vi "Test_StopWatch.vi"() -> ()   [LabVIEW 2018]
panel:
  in  "File":bool
  out "履歴":T1(array[cluster])
  out "FromLap":u32
  out "FromStart":u32
  in  "Lap":bool
  in  "Start":bool
  in  "停止":bool
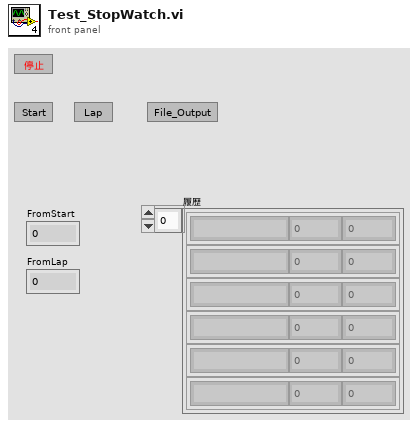
[diagram p1: front panel]
types:
  T1 = cluster{"Point":string, "FromLap":u32, "FromStart":u32}[]
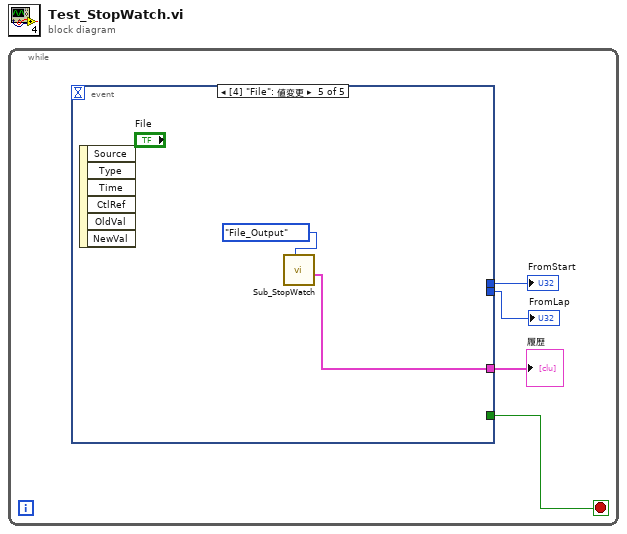
[diagram p0: block diagram]
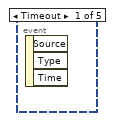
[diagram p2: hidden frame]
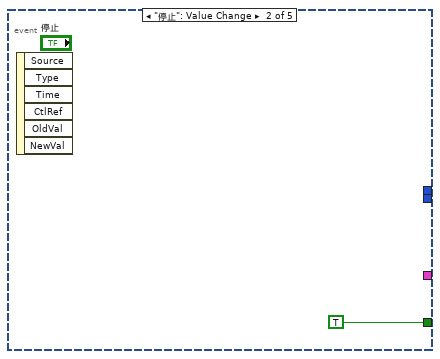
[diagram p3: hidden frame]
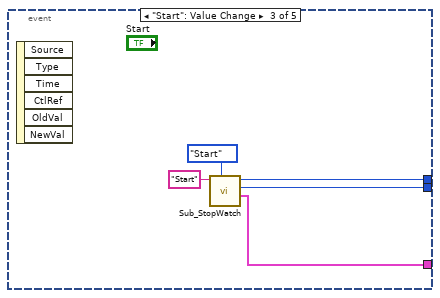
[diagram p4: hidden frame]
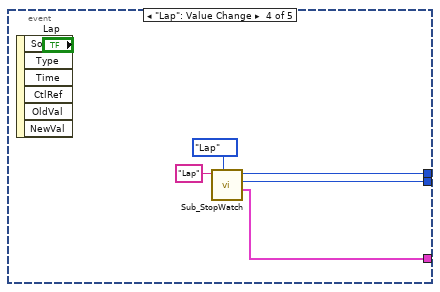
[diagram p5: hidden frame]
diagram:
  n1 = while {
    stop <- w4 stop-if-true
    n2 = event shown="[4] \"File\": 値変更" {
      selector: _ -> [_ _ _ _ _]
      dyn-events: _ -> [_ _ _ _ _]
      timeout: _ -> [_ _ _ _ _]
      tunnel: [_ TRUE _ _ _] -> w4
      tunnel: [_ _ w10 w14 _] -> w3
      tunnel: [_ _ w9 w15 _] -> w2
      tunnel: [_ _ w7 w12 w16] -> w1
      event Timeout {
        n3 = event-data() -> ()  [unwired: 1 in, 3 out]
      }
      event "停止": Value Change {
        n4 = event-data() -> ()  [unwired: 1 in, 6 out]
      }
      event "Start": Value Change {
        n5 = event-data() -> ()  [unwired: 1 in, 6 out]
        n6 = call "Sub_StopWatch.vi"("処理"=enum16{"Start", "Lap", "File_Output"}."Start", "Point"="Start") -> ("履歴"=w7:T1, "FromLap"=w9:u32, "FromStart"=w10:u32)  [unwired: 7 in]
      }
      event "Lap": Value Change {
        n7 = event-data() -> ()  [unwired: 1 in, 6 out]
        n8 = call "Sub_StopWatch.vi"("処理"=enum16{"Start", "Lap", "File_Output"}."Lap", "Point"="Lap") -> ("履歴"=w12:T1, "FromLap"=w15:u32, "FromStart"=w14:u32)  [unwired: 7 in]
      }
      event "File": Value Change {
        n9 = event-data() -> ()  [unwired: 1 in, 6 out]
        n10 = call "Sub_StopWatch.vi"("処理"=enum16{"Start", "Lap", "File_Output"}."File_Output") -> ("履歴"=w16:T1)  [unwired: 8 in, 2 out]
      }
    }
    "FromStart" <- w3
    "FromLap" <- w2
    "履歴" <- w1
  }
